vi "Voltages_2_I16.vi"(0 "Voltages":dbl[][](array[numeric])) -> (1 "Group Channel Settings":T1(array[cluster]), 2 "I16 data":i16[][](array[numeric]))   [LabVIEW 2010]
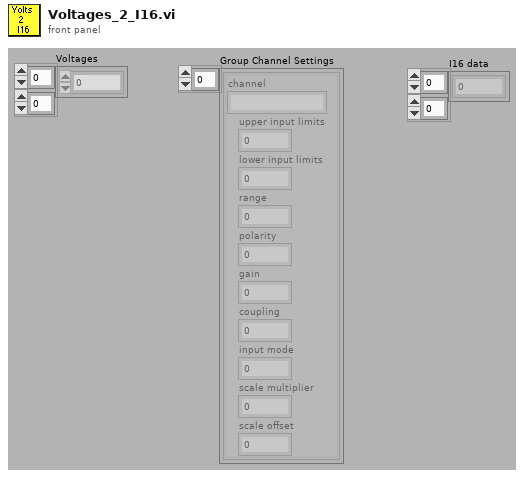
[diagram p1: front panel]
types:
  T1 = cluster{"channel":string, "upper input limits":sgl, "lower input limits":sgl, "range":sgl, "polarity":u16, "gain":sgl, "coupling":u16, "input mode":u16, "scale multiplier":dbl, "scale offset":dbl}[]
  T2 = cluster{"channel":string, "upper input limits":sgl, "lower input limits":sgl, "range":sgl, "polarity":u16, "gain":sgl, "coupling":u16, "input mode":u16, "scale multiplier":dbl, "scale offset":dbl}
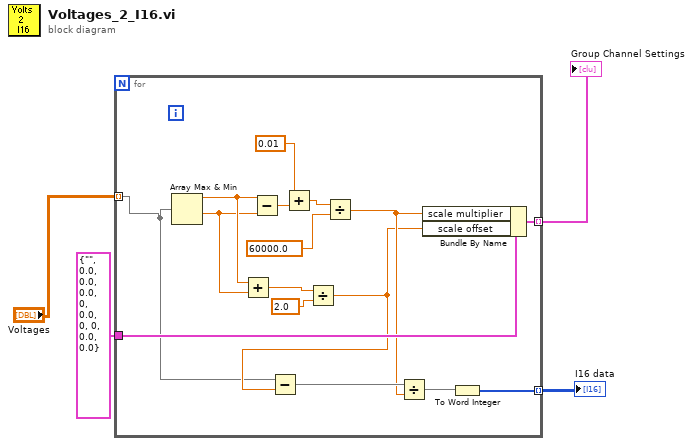
[diagram p0: block diagram]
diagram:
  n1 = for {
    tunnel: T2 {"channel"="", "upper input limits"=0.0, "lower input limits"=0.0, "range"=0.0, "polarity"=0, "gain"=0.0, "coupling"=0, "input mode"=0, "scale multiplier"=0.0, "scale offset"=0.0} -> [w20]
    tunnel: [w19] -> w3 mode=indexing
    tunnel: [w13] -> w2 mode=indexing
    tunnel: "Voltages" -> [w8] mode=indexing
    n2 = Array Max & Min(array=w8) -> (max value=w18:dbl, min value=w17:dbl)  [unwired: 2 out]
    n3 = Add(x=w18, y=w17) -> (x+y=w16:dbl)
    n4 = Subtract(x=w18, y=w17) -> (x-y=w7:dbl)
    n5 = Add(x=0.01, y=w7) -> (x+y=w6:dbl)
    n6 = Divide(x=w16, y=2.0) -> (x/y=w9:dbl)
    n7 = Subtract(x=w8, y=w9) -> (x-y=w11:dbl[])
    n8 = Divide(x=w6, y=60000.0) -> (x/y=w10:dbl)
    n9 = Divide(x=w11, y=w10) -> (x/y=w14:dbl[])
    n10 = Bundle By Name(cluster=w20, "scale multiplier"=w10, "scale offset"=w9) -> (w19:T2)
    n11 = To Word Integer(number=w14) -> (16bit integer=w13:i16[])
  }
  "Group Channel Settings" <- w3
  "I16 data" <- w2
